vi "On_Off_with_hysteresis.vi"(4 "Shift In":dbl[](array[numeric]), 5 "History length":i32=10, 6 "Reset Average after Seconds":dbl=120.0, 7 "New Value":bool) -> (0 "Shift Out":dbl[](array[numeric]), 3 "Output State":bool)   [LabVIEW 2022 SP3]
panel:
  out "mean":dbl format="%0.2f"
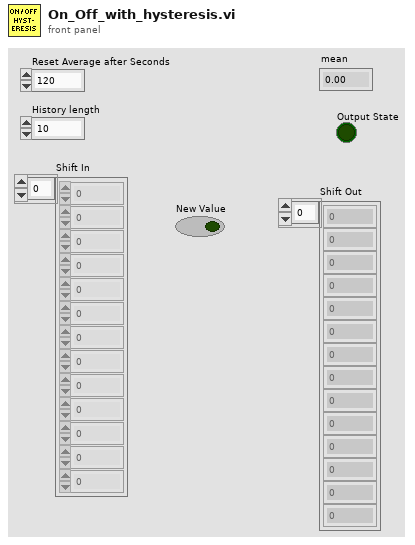
[diagram p1: front panel]
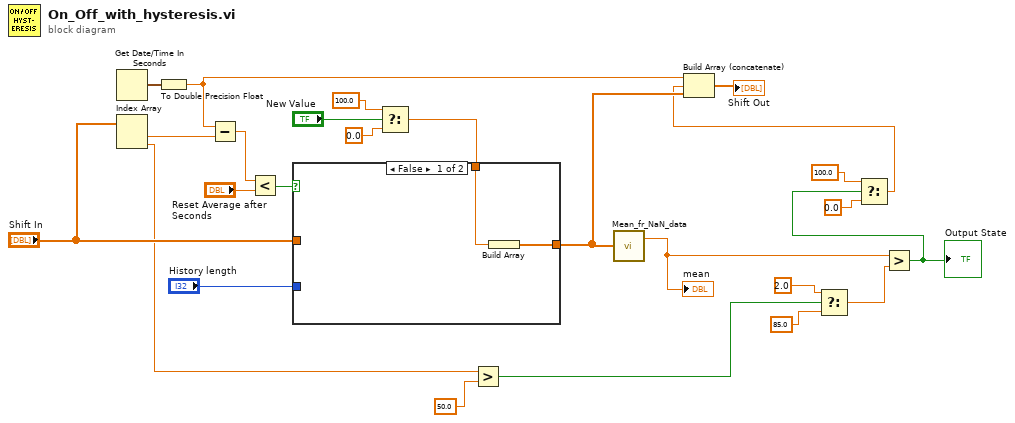
[diagram p0: block diagram]
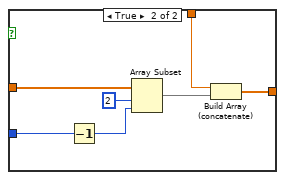
[diagram p2: hidden frame]
diagram:
  n1 = Get Date/Time In Seconds() -> (seconds since 1Jan1904=w25:timestamp)
  n2 = Index Array(array="Shift In") -> (element #1=w24:dbl, element #2=w3:dbl)  [unwired: 2 in]
  n3 = To Double Precision Float(number=w25) -> (double precision float=w12:dbl)
  n4 = Subtract(x=w12, y=w24) -> (x-y=w23:dbl)
  n5 = Less?(x=w23, y="Reset Average after Seconds") -> (x < y?=w21:bool)
  n6 = Select(t=100.0, s="New Value", f=0.0) -> (s? t:f=w13:dbl)
  n7 = case shown="False" w21 {
    tunnel: "Shift In" -> [_ w34]
    tunnel: w13 -> [w27 w28]
    tunnel: [w26 w31] -> w17
    tunnel: "History length" -> [_ w30]
    frame False {
      n8 = Build Array(w27) -> (w26:dbl[])
    }
    frame True {
      n9 = Decrement(x=w30) -> (x-1=w29:i32)
      n10 = Array Subset(array=w34, index=2, length=w29) -> (w32:dbl[])
      n11 = Build Array (concatenate)(w28, w32) -> (w31:dbl[])
    }
  }
  n12 = Greater?(x=w3, y=50.0) -> (0:w1:bool)
  n13 = call "Mean_fr_NaN_data.vi"("Data"=w17) -> ("Mean value"=w11:dbl)  [unwired: 1 out]
  "mean" <- w11
  n14 = Select(t=2.0 ("y"), s=w1, f=85.0 ("y")) -> (s? t:f=w8:dbl)
  n15 = Greater?(x=w11, y=w8) -> (0:w5:bool)
  "Output State" <- w5
  n16 = Select(t=100.0, s=w5, f=0.0) -> (s? t:f=w4:dbl)
  n17 = Build Array (concatenate)(w12, w4, w17) -> (→"Shift Out":dbl[])
